vi "readdosettings.vi"(2 "Path":path, 3 "error in (no error)":errorcluster) -> (5 "Path 2":path, 6 "?":T1, 7 "error out":errorcluster)   [LabVIEW 2012]
uses:
  <vilib>/Utility/config.llb/Read Key (Double).vi
  <vilib>/Utility/config.llb/NI_LVConfig.lvlib
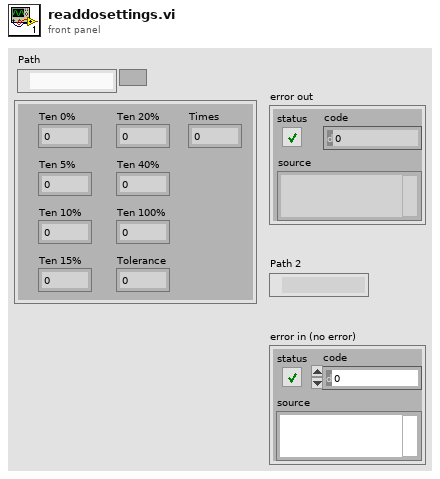
[diagram p1: front panel]
types:
  T1 = cluster{"Ten 0%":dbl, "Ten 5%":dbl, "Ten 10%":dbl, "Ten 15%":dbl, "Tolerance":dbl, "Ten 20%":dbl, "Ten 40%":dbl, "Ten 100%":dbl, "Times":dbl}
  T2 = typedef "NI_LVConfig.lvlib/Config Data RefNum.ctl" = refnum<k1>
  T3 = cluster{"value":dbl, "value":dbl, "value":dbl, "value":dbl, "value":dbl, "value":dbl, "value":dbl, "value":dbl, "value":dbl}
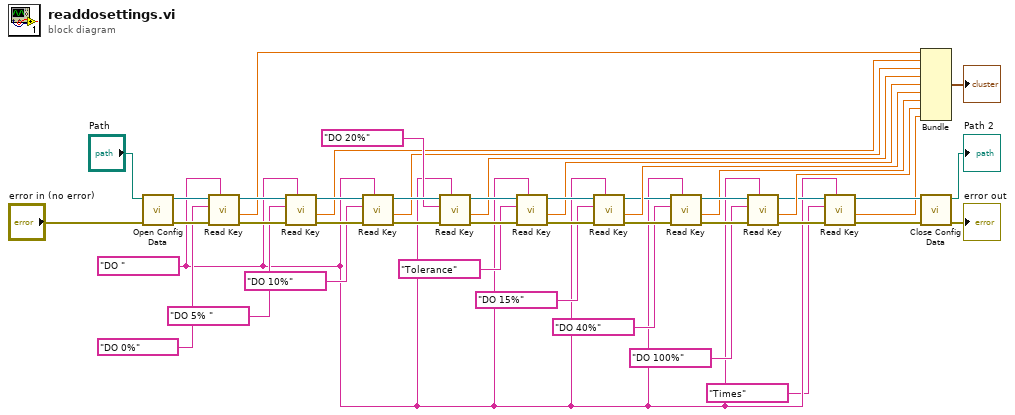
[diagram p0: block diagram]
diagram:
  w4 = "DO "
  n1 = call <vilib>:"Open Config Data.vi"("error in (no error)"="error in (no error)", "configuration file path"="Path") -> ("error out"=w37:errorcluster, "refnum"=w43:T2)  [unwired: 7 in, 1 out]
  n2 = call-poly <vilib>:"Read Key.vi"("section"=w4, "error in (no error)"=w37, "key"="DO 0%", "refnum"=w43) -> ("error out"=w36:errorcluster, "value"=w19:dbl, "refnum out"=w42:T2)  [unwired: 4 in, 1 out]
  n3 = call-poly <vilib>:"Read Key.vi"("section"=w4, "error in (no error)"=w36, "key"="DO 5% ", "refnum"=w42) -> ("error out"=w35:errorcluster, "value"=w20:dbl, "refnum out"=w41:T2)  [unwired: 4 in, 1 out]
  n4 = call-poly <vilib>:"Read Key.vi"("section"=w4, "error in (no error)"=w35, "key"="DO 10%", "refnum"=w41) -> ("error out"=w34:errorcluster, "value"=w21:dbl, "refnum out"=w40:T2)  [unwired: 4 in, 1 out]
  n5 = call-poly <vilib>:"Read Key.vi"("section"=w4, "error in (no error)"=w34, "key"="DO 20%", "refnum"=w40) -> ("error out"=w33:errorcluster, "value"=w22:dbl, "refnum out"=w39:T2)  [unwired: 4 in, 1 out]
  n6 = call-poly <vilib>:"Read Key.vi"("section"=w4, "error in (no error)"=w33, "key"="Tolerance", "refnum"=w39) -> ("error out"=w32:errorcluster, "value"=w23:dbl, "refnum out"=w38:T2)  [unwired: 4 in, 1 out]
  n7 = call-poly <vilib>:"Read Key.vi"("section"=w4, "error in (no error)"=w32, "key"="DO 15%", "refnum"=w38) -> ("error out"=w14:errorcluster, "value"=w24:dbl, "refnum out"=w16:T2)  [unwired: 4 in, 1 out]
  n8 = call-poly <vilib>:"Read Key.vi"("section"=w4, "error in (no error)"=w14, "key"="DO 40%", "refnum"=w16) -> ("error out"=w13:errorcluster, "value"=w1:dbl, "refnum out"=w15:T2)  [unwired: 4 in, 1 out]
  n9 = call-poly <vilib>:"Read Key.vi"("section"=w4, "error in (no error)"=w13, "key"="DO 100%", "refnum"=w15) -> ("error out"=w8:errorcluster, "value"=w12:dbl, "refnum out"=w9:T2)  [unwired: 4 in, 1 out]
  n10 = call-poly <vilib>:"Read Key.vi"("section"=w4, "error in (no error)"=w8, "key"="Times", "refnum"=w9) -> ("error out"=w6:errorcluster, "value"=w5:dbl, "refnum out"=w7:T2)  [unwired: 4 in, 1 out]
  n11 = Bundle("value"=w19, "value"=w20, "value"=w21, "value"=w22, "value"=w23, "value"=w24, "value"=w1, "value"=w12, "value"=w5) -> (→"?":T3)  [unwired: 1 in]
  n12 = call <vilib>:"Close Config Data.vi"("error in (no error)"=w6, "refnum"=w7) -> ("error out"=→"error out":errorcluster, "file path"=→"Path 2":path)  [unwired: 8 in]
